vi "line profile.vi"(7 "error in":errorcluster) -> (27 "error out":errorcluster)   [LabVIEW 2009]
uses:
  <vilib>/vision/NI_Vision_Development_Module.lvlib
panel:
  out "Image Out":T1(plugin-control)
  out "Line Profile Graph 2":cluster{"x0":sgl, "dx":sgl, "Pixels Line":sgl[]}(graph) caption="Line Profile"
  out "Line Profile Graph":cluster{"x0":sgl, "dx":sgl, "Pixels Line":sgl[]}(graph) caption="Line Profile"
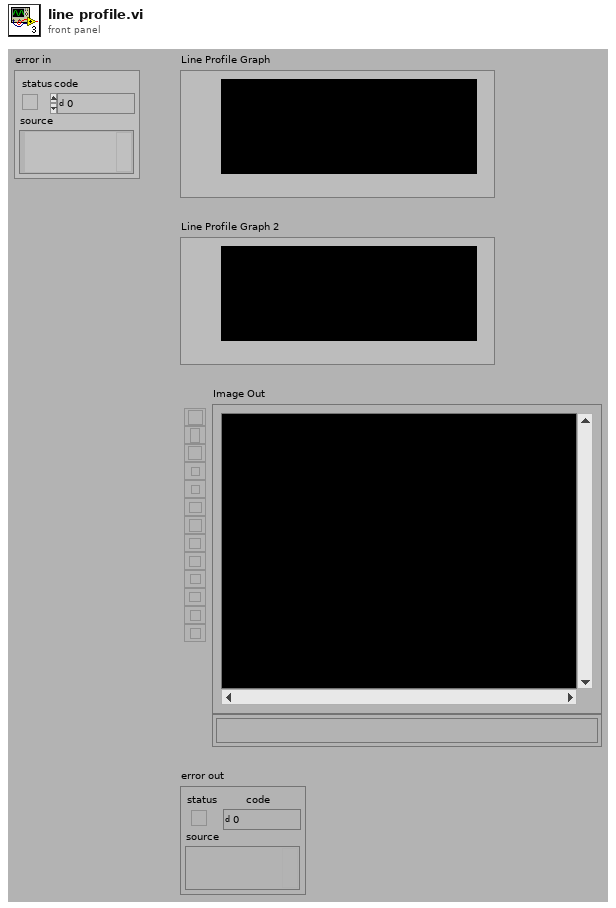
[diagram p1: front panel]
types:
  T1 = typedef "IMAQ Image.ctl" = refnum<image>
  T2 = cluster{"Global Rectangle":i32[], "Contours":cluster{"ID":enum32{"External", "Internal"}, "Type":u32, "Coordinates":i32[]}[]}
  T3 = cluster{"Min":sgl, "Max":sgl, "Mean":sgl, "Std Dev":sgl, "Count":i32}
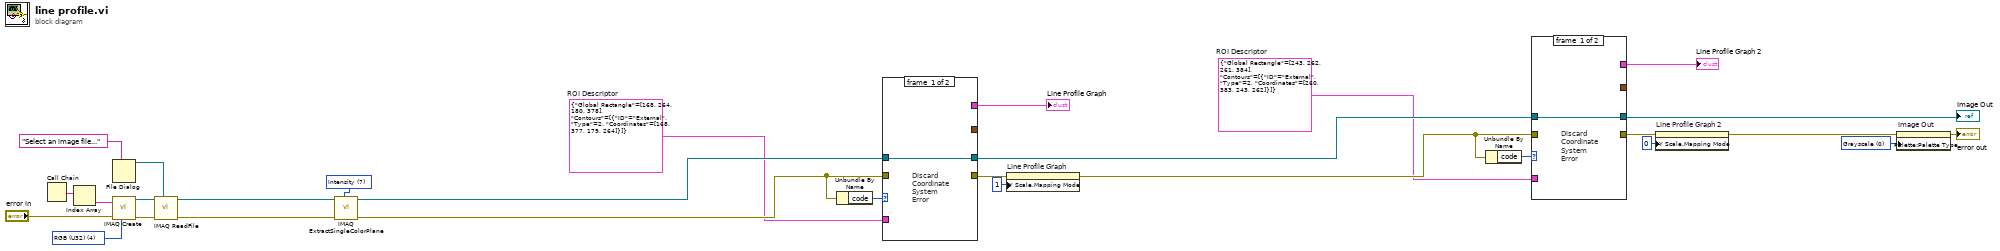
[diagram p0: block diagram]
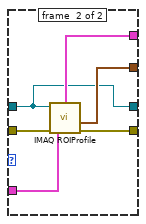
[diagram p2: hidden frame]
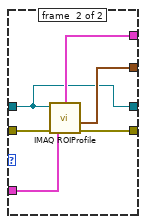
[diagram p3: hidden frame]
diagram:
  w2 = u32 0 items=["Grayscale", "Binary", "Gradient", "Rainbow", "Temperature", "User Defined"] ("Palette")
  w5 = T2 {"Global Rectangle"=[243, 262, 261, 384], "Contours"=[{"ID"=enum."External", "Type"=2, "Coordinates"=[260, 383, 243, 262]}]}  # ROI Descriptor
  w12 = T2 {"Global Rectangle"=[168, 264, 180, 378], "Contours"=[{"ID"=enum."External", "Type"=2, "Coordinates"=[168, 377, 179, 264]}]}  # ROI Descriptor
  w20 = 7 items=["Red", "Green", "Blue", "Hue", "Saturation", "Luminance", "Value", "Intensity"] ("Color Plane")
  w26 = u32 4 items=["Grayscale (U8)", "Grayscale (I16)", "Grayscale (SGL)", "Complex (CSG)", "RGB (U32)", "HSL (U32)", "RGB (U64)"] ("Image Type")
  n1 = Call Chain() -> (call chain=w22:string[])
  n2 = Index Array(array=w22) -> (element=w21:string)  [unwired: 1 in]
  n3 = File Dialog(7:"Select an image file..." ("prompt")) -> (3:w25:path)  [unwired: 1 in, 8 out]
  n4 = call "IMAQ Create"("Image Name"=w21, "Image Type"=w26, "error in (no error)"="error in") -> ("New Image"=w28:T1, "error out"=w27:errorcluster)  [unwired: 1 in, 1 out]
  n5 = call "IMAQ ReadFile"("File Path"=w25, "error in (no error)"=w27, "Image"=w28) -> ("error out"=w29:errorcluster, "Image Out"=w19:T1)  [unwired: 2 in, 5 out]
  n6 = call "IMAQ ExtractSingleColorPlane"("Color Plane"=w20, "error in (no error)"=w29, "Image Src"=w19) -> ("error out"=w18:errorcluster, "Image Dst Out"=w14:T1)  [unwired: 1 in, 6 out]
  n7 = Unbundle By Name(w18) -> ("code"=w11:i32)
  n8 = case shown="Default" w11 {
    tunnel: w18 -> [_ w36]
    tunnel: [_ w35] -> _
    tunnel: [_ w34] -> w16
    tunnel: w14 -> [w30 w31]
    tunnel: [_ w33] -> w13
    tunnel: w12 -> [_ w32]
    tunnel: [w30 w31] -> w7
    frame #0 {
      # "Discard\nCoordinate\nSystem\nError"
    }
    frame #1 {
      n9 = call "IMAQ ROIProfile"("error in (no error)"=w36, "ROI Descriptor"=w32, "Image"=w31) -> ("ROI Pixel Statistics"=w35:T3, "error out"=w34:errorcluster, "ROI Graph"=w33:cluster{"x0":sgl, "dx":sgl, "Pixels Line":sgl[]})  [unwired: 3 out]
    }
  }
  "Line Profile Graph" <- w13
  n10 = property on="Line Profile Graph" class="WFGraph"(error in=w16, "Y Scale.Mapping Mode"=u8 1) -> (error out=w15:errorcluster)  [unwired: 1 in, 1 out]
  n11 = Unbundle By Name(w15) -> ("code"=w4:i32)
  n12 = case shown="Default" w4 {
    tunnel: w15 -> [_ w43]
    tunnel: [_ w42] -> _
    tunnel: [_ w41] -> w9
    tunnel: w7 -> [w37 w38]
    tunnel: [_ w40] -> w6
    tunnel: w5 -> [_ w39]
    tunnel: [w37 w38] -> w3
    frame #0 {
      # "Discard\nCoordinate\nSystem\nError"
    }
    frame #1 {
      n13 = call "IMAQ ROIProfile"("error in (no error)"=w43, "ROI Descriptor"=w39, "Image"=w38) -> ("ROI Pixel Statistics"=w42:T3, "error out"=w41:errorcluster, "ROI Graph"=w40:cluster{"x0":sgl, "dx":sgl, "Pixels Line":sgl[]})  [unwired: 3 out]
    }
  }
  "Line Profile Graph 2" <- w6
  "Image Out" <- w3
  n14 = property on="Line Profile Graph 2" class="WFGraph"(error in=w9, "Y Scale.Mapping Mode"=u8 0) -> (error out=w8:errorcluster)  [unwired: 1 in, 1 out]
  n15 = property on="Image Out" class="ImageControl"(error in=w8, "Palette:Palette Type"=w2) -> (error out=→"error out":errorcluster)  [unwired: 1 in, 1 out]
